vi "Get JSON Config Value.vi"(7 "Data Value ID":string, 11 "Test in":refnum<class "Test.lvclass">) -> (2 "Data Value":string)   [LabVIEW 2018, in "Test.lvclass"]
uses:
  Test.lvclass
  Test.lvclass/Test.ctl
  <vilib>/JDP Science/JSONtext/String Subset.vi
  <vilib>/JDP Science/JSONtext/Parsing/Parse Full Path or Item Name.vi
  <vilib>/JDP Science/JSONtext/Offset/Find Item Locations by Path.vi
  <vilib>/JDP Science/JSONtext/JSONtext.lvlib
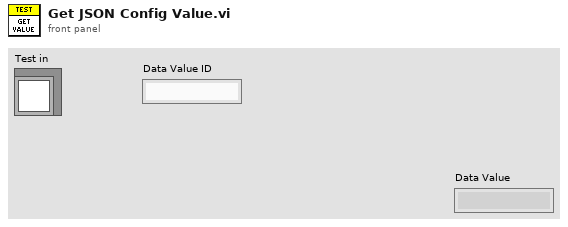
[diagram p1: front panel]
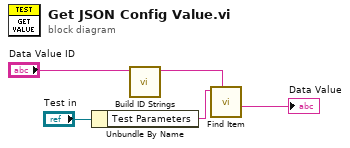
[diagram p0: block diagram]
diagram:
  n1 = Unbundle By Name("Test in") -> ("Test Parameters"=w4:string)
  n2 = call "Build ID Strings.vi"("Data Value ID"="Data Value ID") -> ("Value ID"=w2:string)  [unwired: 9 in, 1 out]
  n3 = call <vilib>:"Find Item.vi"("$Path or Item Name"=w2, "JSON"=w4) -> ("<JSON>"=→"Data Value":string)  [unwired: 6 in, 3 out]
